vi "Tell Parent.vi"(4 "Priority":bool, 7 "Actor in":refnum<class "Actor.lvclass">, 8 "Error in":errorcluster, 10 "Msg":refnum<class "Msg.lvclass">) -> (0 "Error out":errorcluster, 5 "Actor out":refnum<class "Actor.lvclass">)   [LabVIEW 2025, in "jettl.lvlib"]
uses:
  jettl.lvlib
  Relation.ctl
  Actor/Actor.lvclass
  Attributes/Attributes.lvclass
  Transport/Transport.lvclass
  Msg/Msg.lvclass
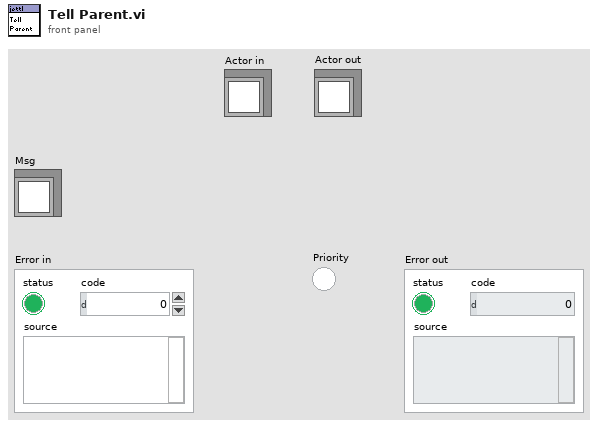
[diagram p1: front panel]
types:
  T1 = typedef "jettl.lvlib/Relation.ctl" = enum16{"Self", "Parent", "Child", "No Relation"}
  T2 = typedef "jettl.lvlib/Msgs.ctl" = set{refnum<class "Msg.lvclass">}
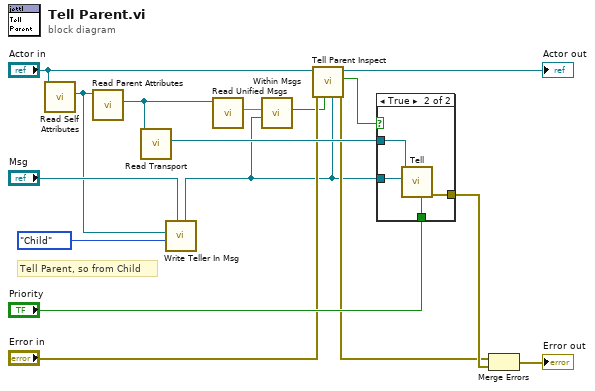
[diagram p0: block diagram]
diagram:
  # "Tell Parent, so from Child"
  n1 = call-dynamic "Read Self Attributes.vi"("Actor in"="Actor in") -> ("Self Attributes"=w6:refnum<class "Attributes.lvclass">)  [unwired: 10 in]
  n2 = call-dynamic "Read Parent Attributes.vi"("Attributes in"=w6) -> ("Parent Attributes"=w4:refnum<class "Attributes.lvclass">)  [unwired: 10 in]
  n3 = call-dynamic "Read Transport.vi"("Attributes in"=w4) -> ("Transport"=w15:refnum<class "Transport.lvclass">)  [unwired: 10 in]
  n4 = call "Write Teller In Msg.vi"("Msg in"="Msg", "Relation"=Relation."Child", "Attributes"=w6) -> ("Msg out"=w2:refnum<class "Msg.lvclass">)  [unwired: 8 in]
  n5 = call-dynamic "Read Unified Msgs.vi"("Attributes in"=w4) -> ("Unified Msgs"=w5:T2)  [unwired: 10 in]
  n6 = call "Within Msgs.vi"("Msg"=w2, "Msgs"=w5) -> ("Within Msgs"=w3:bool)  [unwired: 9 in]
  n7 = call-dynamic "Tell Parent Inspect.vi"("Msg"=w2, "Within Unified Msgs"=w3, "Error in"="Error in", "Actor in"="Actor in") -> ("Error out"=w7:errorcluster, "Proceed"=w1:bool, "Actor out"=→"Actor out":refnum<class "Actor.lvclass">)  [unwired: 5 in]
  n8 = case shown="True" w1 {
    tunnel: [_ w20] -> w16
    tunnel: w15 -> [_ w19]
    tunnel: "Priority" -> [_ w18]
    tunnel: w2 -> [_ w17]
    frame False {
    }
    frame True {
      n9 = call-dynamic "Tell.vi"("Priority"=w18, "Msg"=w17, "Transport in"=w19) -> ("Error out"=w20:errorcluster)  [unwired: 8 in]
    }
  }
  n10 = Merge Errors(w7, w16) -> (→"Error out":errorcluster)
